vi "Manual.vi"(6 "Cluster":T8={"VISA resource name"="", "baud rate "=9600}, 7 "vi reference":refnum<vi>, 8 "error in (no error)":errorcluster, 9 "IOList_280":T1, 11 "Manual":T4(tab)) -> (0 "error out":errorcluster, 3 "Out reference":refnum<vi>)   [LabVIEW 2015]
uses:
  Control Button/Exit.ctl
  Control Button/Scanner config.ctl
  Galobal variable_TI.vi
  <vilib>/Instr/_visa.llb/VISA Configure Serial Port (Instr).vi
panel:
  out "Z Dir Dn":bool
  out "Z dir Up":bool
  out "Screw SlideFWD":bool
  out "Screw SlideRev":bool
  out "Array":string[](array[string])
  out "Byte Lenth":i32
  out "error out 2":errorcluster
  in  "Stop":T2
  out "NewVal":T3
  in  "Digital Output":T5
  out "LVDT":string
  out "Digital Input":T6
  out "Error Message":string
  out "Dist. data":dbl[](array[numeric]) format="%0.03f"
  out "Error Status":bool
  in  "Scanner config":T7
  out "Read data":string
  out "Boolean":bool
  # "Instruction for Servo motor Operate\n(1)  Switch  ON -OFF  of Fixture Slide servo Brake ON Cmd (P0.19)  \n      from Digital Output tab.\n(2) Switch  ON -OFF  of Fixture Slide Servo Direction Command (P0.20)\n      from Digital Output tab."
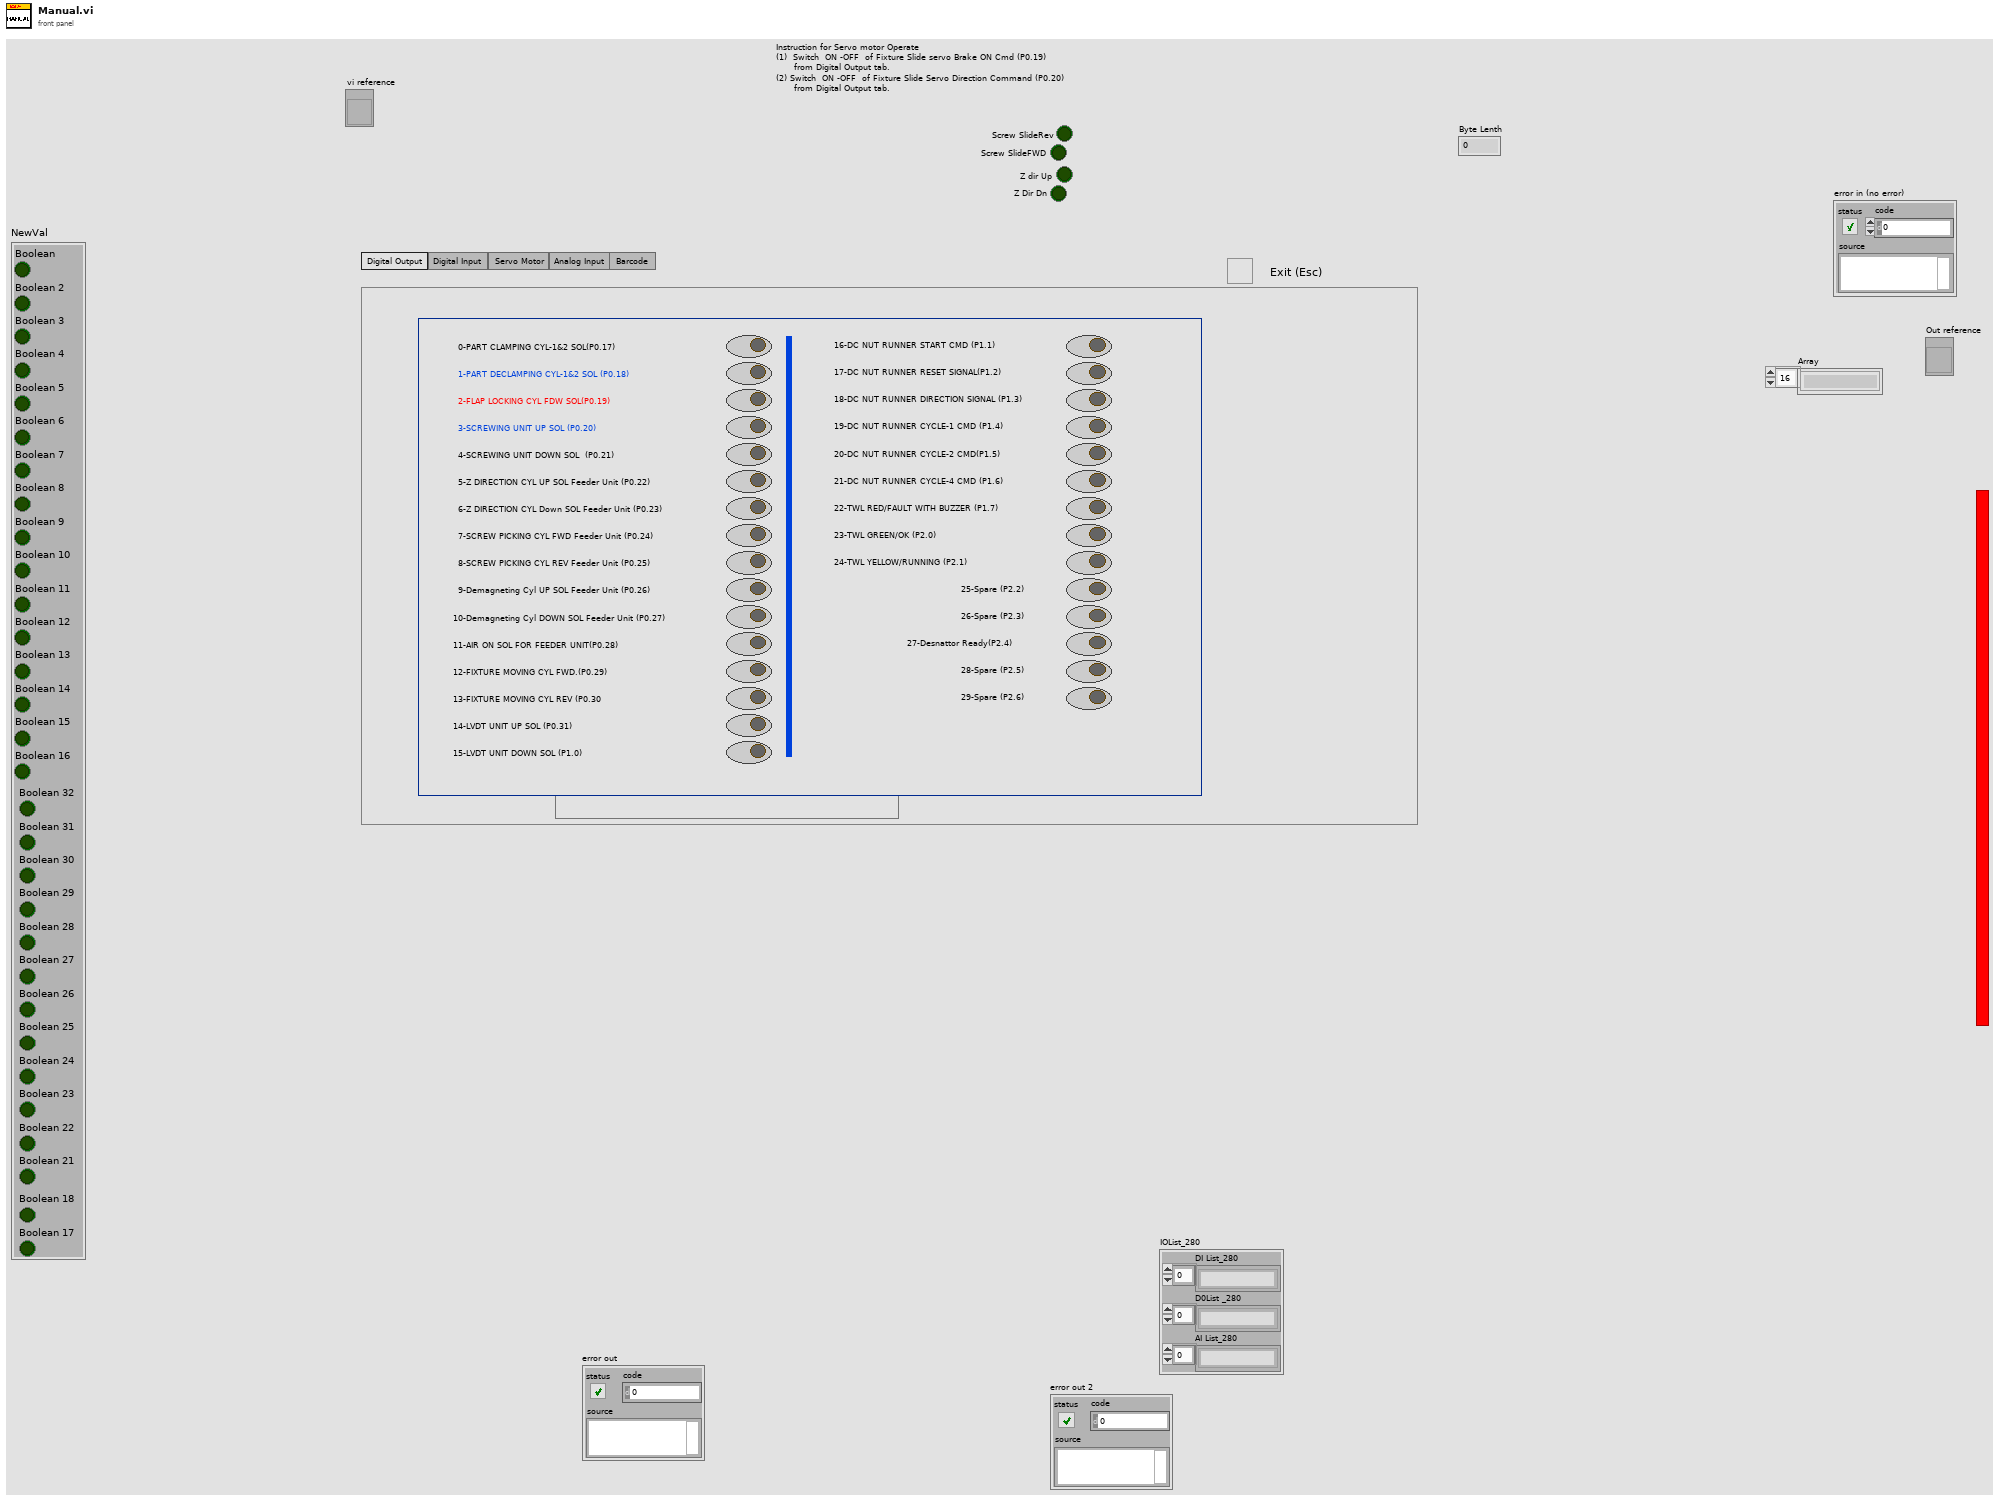
[diagram p1: front panel]
types:
  T1 = cluster{"DI List_280":string[], "D0List _280":string[], "AI List_280":string[]}
  T2 = typedef "Exit.ctl" = bool
  T3 = cluster{"Boolean":bool, "Boolean 2":bool, "Boolean 3":bool, "Boolean 4":bool, "Boolean 5":bool, "Boolean 6":bool, "Boolean 7":bool, "Boolean 8":bool, "Boolean 9":bool, "Boolean 10":bool, "Boolean 11":bool, "Boolean 12":bool, "Boolean 13":bool, "Boolean 14":bool, "Boolean 15":bool, "Boolean 16":bool, "Boolean 17":bool, "Boolean 18":bool, "Boolean 21":bool, "Boolean 22":bool, "Boolean 23":bool, "Boolean 24":bool, "Boolean 25":bool, "Boolean 26":bool, "Boolean 27":bool, "Boolean 28":bool, "Boolean 29":bool, "Boolean 30":bool, "Boolean 31":bool, "Boolean 32":bool}
  T4 = enum32{"Digital Output", "Digital Input", "Servo Motor ", "Analog Input", "Barcode "}
  T5 = cluster{"DO.00":bool, "DO.01":bool, "DO.02":bool, "DO.03":bool, "DO.04":bool, "DO.05":bool, "DO.06":bool, "DO.06":bool, "DO.07":bool, "DO.08":bool, "DO.09":bool, "DO.10":bool, "DO.11":bool, "DO.12":bool, "DO.13":bool, "DO.14":bool, "DO.07 2":bool, "DO.08 2":bool, "DO.09 2":bool, "DO.10 2":bool, "DO.11 2":bool, "DO.12 2":bool, "DO.13 2":bool, "DO.14 2":bool, "DO.00 2":bool, "DO.01 2":bool, "DO.02 2":bool, "DO.03 2":bool, "DO.06 2":bool, "DO.06 3":bool}
  T6 = cluster{"Digital Input":bool, "Digital Input 2":bool, "Digital Input 3":bool, "Digital Input 4":bool, "Digital Input 5":bool, "Digital Input 6":bool, "Digital Input 7":bool, "Digital Input 8":bool, "Digital Input 9":bool, "Digital Input 10":bool, "Digital Input 11":bool, "Digital Input 12":bool, "Digital Input 13":bool, "Digital Input 14":bool, "Digital Input 15":bool, "Digital Input 16":bool, "Digital Input 17":bool, "Digital Input 18":bool, "Digital Input 19":bool, "Digital Input 20":bool, "Digital Input 21":bool, "Digital Input 22":bool, "Digital Input 23":bool, "Digital Input 24":bool, "Digital Input 25":bool, "Digital Input 26":bool, "Digital Input 27":bool, "Digital Input 28":bool, "Digital Input 29":bool, "Digital Input 30":bool, "Digital Input 31":bool, "Digital Input 32":bool, "Digital Input 33":bool, "Digital Input 34":bool, "Digital Input 35":bool, "Digital Input 36":bool, "Digital Input 37":bool, "Digital Input 38":bool, "Digital Input 39":bool, "Digital Input 40":bool, "Digital Input 41":bool, "Digital Input 42":bool, "Digital Input 43":bool, "Digital Input 44":bool}
  T7 = typedef "Scanner config.ctl" = bool
  T8 = cluster{"VISA resource name":refnum<visa-resource-name>, "baud rate ":u32}
  T9 = cluster{"Emergency_1":bool, "Reset_2":bool, "Air Pressure_4":bool, "Safety Sensor_5":bool, "Safety Sensor_6":bool, "Barcode Rev rs_24":bool, "Clamp fwd rs_21":bool, "Servo Fault":bool, "Home _3":bool}
  T10 = cluster{"Digital input[0]":bool, "Digital input[1]":bool, "Digital input[2]":bool, "Digital input[3]":bool, "Digital input[4]":bool, "Digital input[5]":bool, "Digital input[6]":bool, "Digital input[7]":bool, "Digital input[8]":bool, "Digital input[9]":bool, "Digital input[10]":bool, "Digital input[11]":bool, "Digital input[12]":bool, "Digital input[13]":bool, "Digital input[14]":bool, "Digital input[15]":bool, "Digital input[16]":bool, "Digital input[17]":bool, "Digital input[18]":bool, "Digital input[19]":bool, "Digital input[20]":bool, "Digital input[21]":bool, "Digital input[22]":bool, "Digital input[23]":bool, "Digital input[24]":bool, "Digital input[25]":bool, "Digital input[26]":bool, "Digital input[27]":bool, "Digital input[28]":bool, "Digital input[29]":bool, "Digital input[30]":bool, "Digital input[31]":bool, "Digital input[32]":bool, "Digital input[33]":bool, "Digital input[34]":bool, "Digital input[35]":bool, "Digital input[36]":bool, "Digital input[37]":bool, "Digital input[38]":bool, "Digital input[39]":bool, "Digital input[40]":bool, "Digital input[41]":bool, "Digital input[42]":bool, "Digital input[43]":bool}
  T11 = enum16{"Z Dir Up  Screw Slide Rev Cyl_Ddir Dn & Up", "Z Dir Dn Cyl Screw Slide Fwd Cyl"}
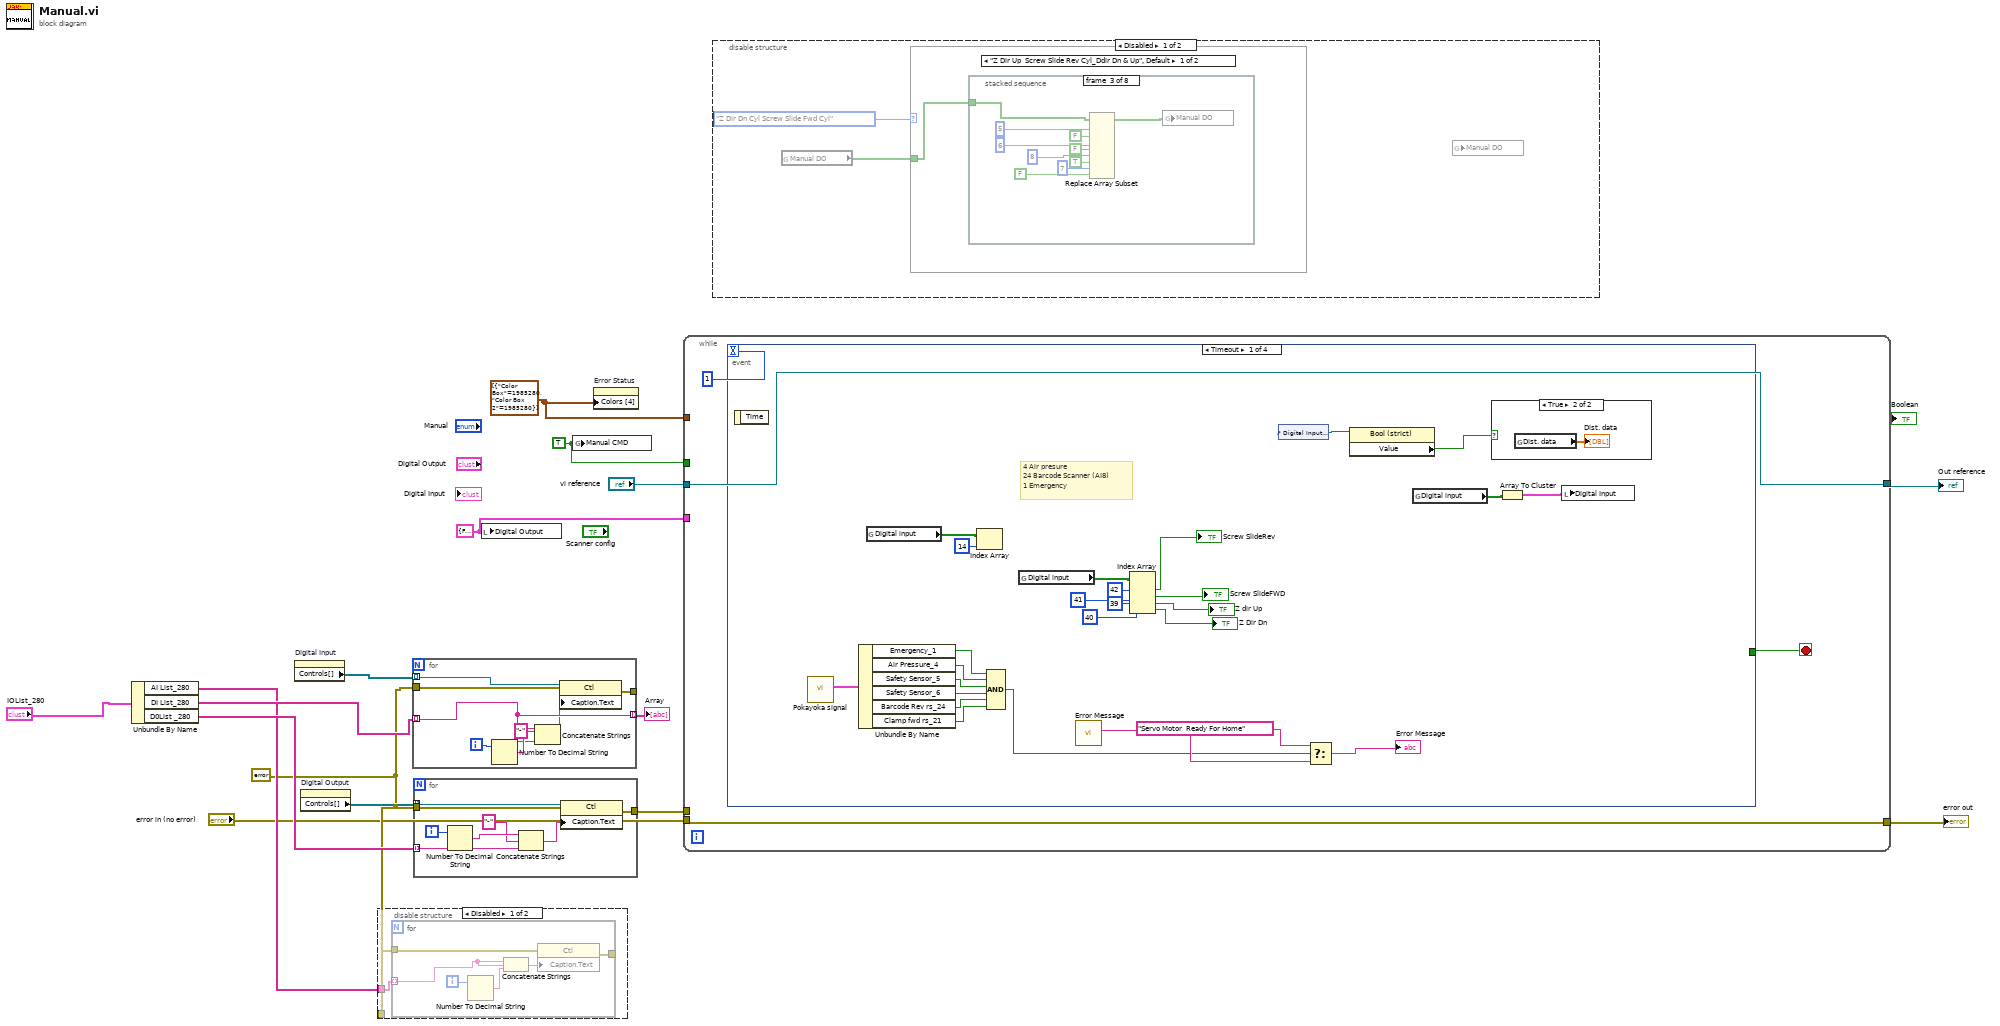
[diagram p0: block diagram]
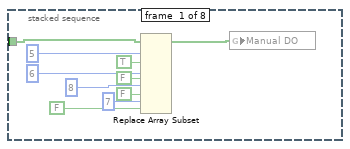
[diagram p2: hidden frame]
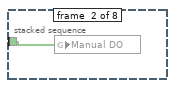
[diagram p3: hidden frame]
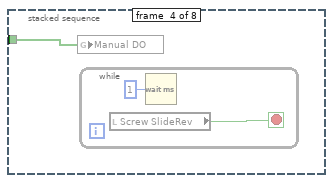
[diagram p4: hidden frame]
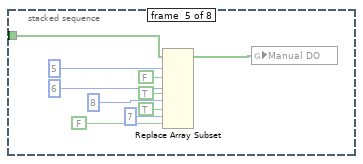
[diagram p5: hidden frame]
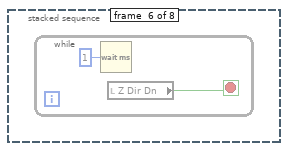
[diagram p6: hidden frame]
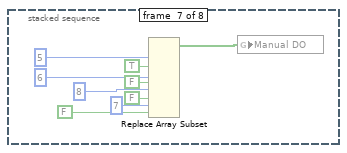
[diagram p7: hidden frame]
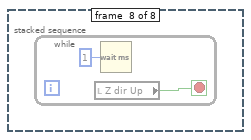
[diagram p8: hidden frame]
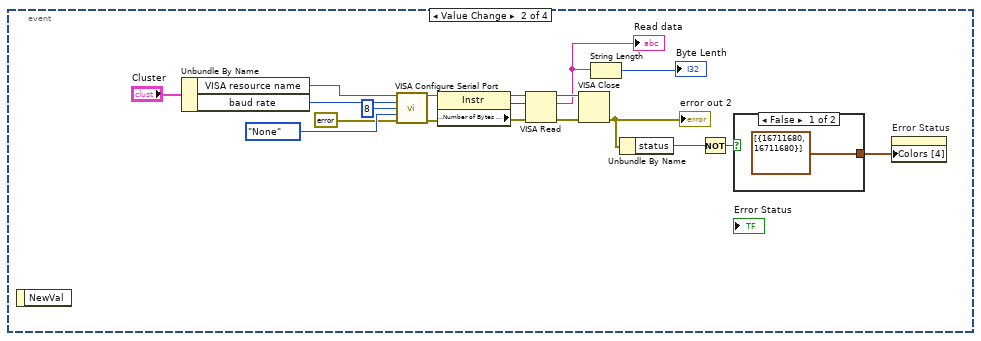
[diagram p13: hidden frame]
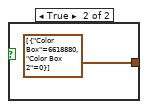
[diagram p14: hidden frame]
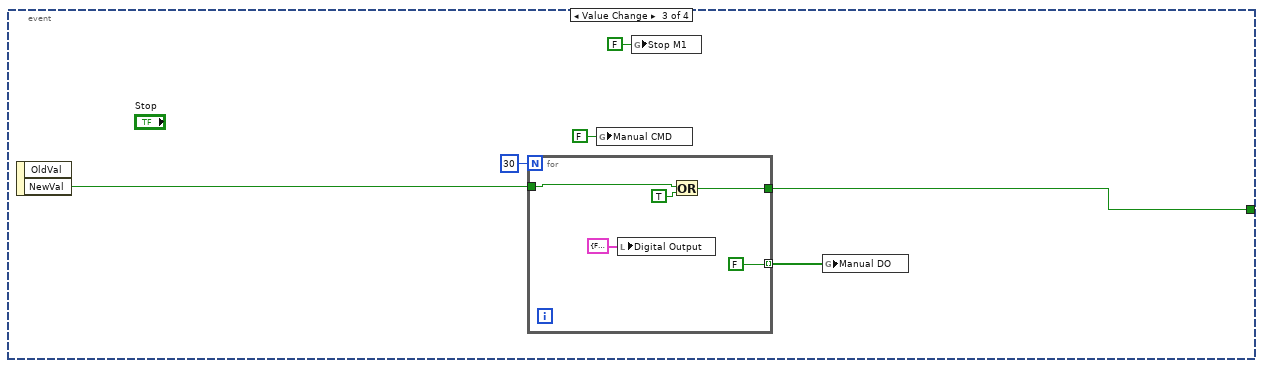
[diagram p15: hidden frame]
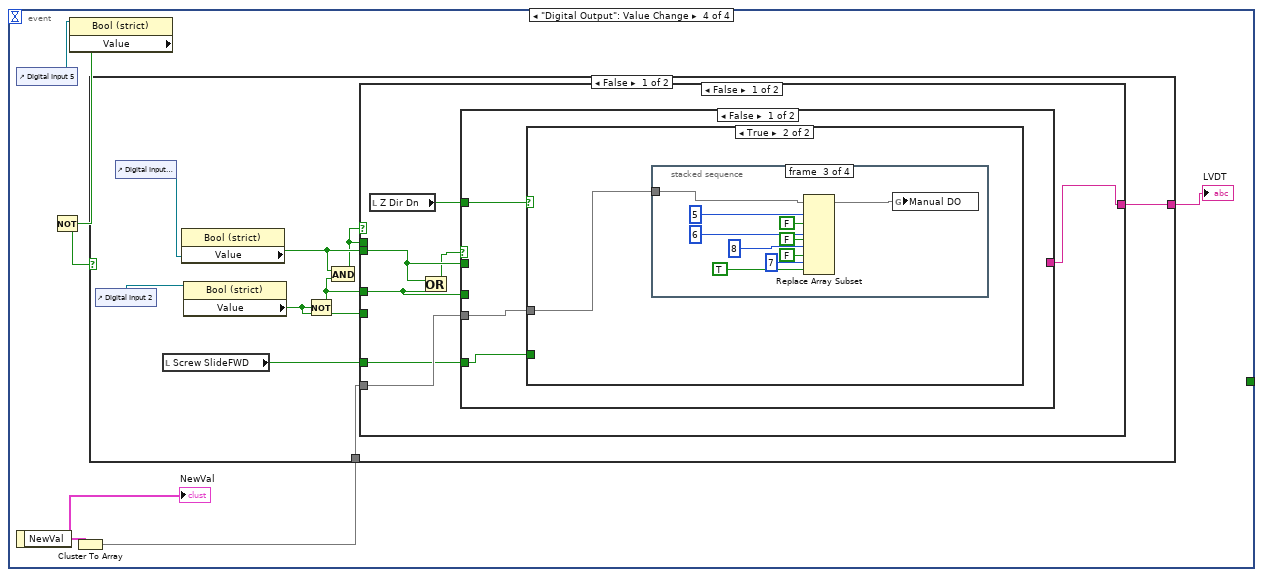
[diagram p16: hidden frame]
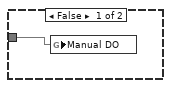
[diagram p17: hidden frame]
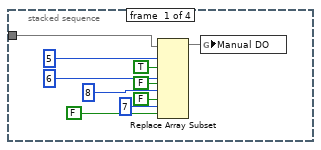
[diagram p18: hidden frame]
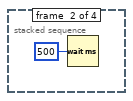
[diagram p19: hidden frame]
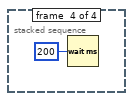
[diagram p20: hidden frame]
diagram:
  w1 = T5 {"DO.00"=FALSE, "DO.01"=FALSE, "DO.02"=FALSE, "DO.03"=FALSE, "DO.04"=FALSE, "DO.05"=FALSE, "DO.06"=FALSE, "DO.06"=FALSE, "DO.07"=FALSE, "DO.08"=FALSE, "DO.09"=FALSE, "DO.10"=FALSE, "DO.11"=FALSE, "DO.12"=FALSE, "DO.13"=FALSE, "DO.14"=FALSE, "DO.07 2"=FALSE, "DO.08 2"=FALSE, "DO.09 2"=FALSE, "DO.10 2"=FALSE, "DO.11 2"=FALSE, "DO.12 2"=FALSE, "DO.13 2"=FALSE, "DO.14 2"=FALSE, "DO.00 2"=FALSE, "DO.01 2"=FALSE, "DO.02 2"=FALSE, "DO.03 2"=FALSE, "DO.06 2"=FALSE, "DO.06 3"=FALSE} ("Digital Output")
  w4 = errorcluster {"status"=FALSE, "code"=0, "source"=""} ("error in (no error)")
  w7 = cluster{"Color Box":u32, "Color Box 2":u32}[] [{"Color Box"=1985280, "Color Box 2"=1985280}] ("Colors [4]")
  w12 = TRUE ("Manual CMD")
  n1 = Unbundle By Name("IOList_280") -> ("AI List_280"=w8:string[], "DI List_280"=w9:string[], "D0List _280"=w11:string[])
  n2 = property on="Digital Input" class="Clust (strict)"() -> ("Controls[]"=w10:refnum<vi>[])  [unwired: 2 in, 2 out]
  n3 = property on="Digital Output" class="Clust (strict)"() -> ("Controls[]"=w15:refnum<vi>[])  [unwired: 2 in, 2 out]
  n4 = disable-structure shown="Disabled" {
    disable-tunnel: w8 -> [w18 _]
    disable-tunnel: w4 -> [w17 _]
    frame Disabled {
      n5 = for {
        tunnel: [w22] -> _
        tunnel: w17 -> [w20]
        tunnel: w18 -> [w19] mode=indexing
        i -> [w23]
        n6 = Number To Decimal String(number=w23) -> (decimal integer string=w21:string)  [unwired: 1 in]
        n7 = Concatenate Strings(w19, w21) -> ()  [unwired: 1 out]
        n8 = property class="Ctl"(error in=w20, "Caption.Text"=w19) -> (error out=w22:errorcluster)  [unwired: 1 in, 1 out]
      }
    }
    frame Enabled {
    }
  }
  n9 = for {
    tunnel: w10 -> [w31] mode=indexing
    tunnel: [w29] -> _
    tunnel: w4 -> [w28]
    tunnel: w9 -> [w25] mode=indexing
    tunnel: [w25] -> w5 mode=indexing
    i -> [w30]
    n10 = Number To Decimal String(number=w30) -> (decimal integer string=w27:string)  [unwired: 1 in]
    n11 = Concatenate Strings(w27, "-" ("string"), w25) -> (w24:string)
    n12 = property class="Ctl"(reference=w31, error in=w28, "Caption.Text"=w24) -> (error out=w29:errorcluster)  [unwired: 1 out]
  }
  "Array" <- w5
  n13 = for {
    tunnel: w15 -> [w39] mode=indexing
    tunnel: [w37] -> w16
    tunnel: w4 -> [w36]
    tunnel: w11 -> [w33] mode=indexing
    i -> [w38]
    n14 = Number To Decimal String(number=w38) -> (decimal integer string=w35:string)  [unwired: 1 in]
    n15 = Concatenate Strings(w35, "-" ("string"), w33) -> (w32:string)
    n16 = property class="Ctl"(reference=w39, error in=w36, "Caption.Text"=w32) -> (error out=w37:errorcluster)  [unwired: 1 out]
  }
  n17 = local write "Digital Output"(w1) -> ()
  n18 = global write "Galobal variable_TI.vi" "Manual CMD"(w12) -> ()
  n19 = property on="Error Status" class="Bool (strict)"("Colors [4]"=w7) -> ()  [unwired: 2 in, 2 out]
  n20 = while {
    tunnel: w16 -> [_]
    tunnel: [w41] -> w14
    tunnel: "vi reference" -> [w42]
    tunnel: [w42] -> w13
    tunnel: w12 -> [_]
    tunnel: w7 -> [_]
    tunnel: "error in (no error)" -> [w41]
    tunnel: w1 -> [_]
    stop <- w40 stop-if-true
    n21 = event shown="[0] Timeout" {
      selector: _ -> [_ _ _ _]
      dyn-events: _ -> [_ _ _ _]
      timeout: 1 -> [_ _ _ _]
      tunnel: [_ _ w92 _] -> w40
      event Timeout {
        # "4 Air presure\n24 Barcode Scanner (AI8)\n1 Emergency"
        n22 = event-data() -> ()  [unwired: 1 in, 1 out]
        n23 = call "Pokayoka signal.vi"() -> ("output cluster"=w64:T9)  [unwired: 10 in, 1 out]
        n24 = Unbundle By Name(w64) -> ("Emergency_1"=w57:bool, "Air Pressure_4"=w63:bool, "Safety Sensor_5"=w62:bool, "Safety Sensor_6"=w61:bool, "Barcode Rev rs_24"=w60:bool, "Clamp fwd rs_21"=w59:bool)
        n25 = global read "Galobal variable_TI.vi" "Digital input"() -> (w56:bool[])
        n26 = Index Array(array=w56, index=14) -> ()  [unwired: 1 out]
        n27 = Compound Arithmetic op=AND(w57, w63, w62, w61, w60, w59) -> (w58:bool)
        n28 = global read "Galobal variable_TI.vi" "Digital input"() -> (w53:bool[])
        n29 = call "Error Message.vi"() -> ("Error"=w66:string)  [unwired: 11 in]
        n30 = Index Array(array=w53, index #1=42 ("index"), index #2=41 ("index"), index #3=39 ("index"), index #4=40 ("index")) -> (element #1=→"Screw SlideRev":bool, element #2=→"Screw SlideFWD":bool, element #3=→"Z dir Up":bool, element #4=→"Z Dir Dn":bool)
        n31 = control-ref of="Digital Input 16"() -> (w45:refnum<vi>)
        n32 = Select(t="Servo Motor  Ready For Home", s=w58, f=w66) -> (s? t:f=→"Error Message":string)
        n33 = property class="Bool (strict)"(reference=w45) -> ("Value"=w44:bool)  [unwired: 1 in, 2 out]
        n34 = global read "Galobal variable_TI.vi" "Digital input"() -> (w68:bool[])
        n35 = case shown="True" w44 {
          frame False {
          }
          frame True {
            n36 = global read "Galobal variable_TI.vi" "Dist. data"() -> (→"Dist. data":dbl[])
          }
        }
        n37 = Array To Cluster(array=w68) -> (cluster=w69:T10)
        n38 = local write "Digital Input"(w69) -> ()
      }
      event Value Change {
        n39 = event-data() -> ()  [unwired: 1 in, 1 out]
        n40 = Unbundle By Name("Cluster") -> ("VISA resource name"=w89:refnum<visa-resource-name>, "baud rate"=w88:u32)
        n41 = call-poly "VISA Configure Serial Port"("VISA resource name"=w89, "baud rate (9600)"=w88, "data bits (8)"=u16 8, "parity (0:none)"=enum16{"None", "Odd", "Even", "Mark", "Space"}."None", "error in (no error)"=errorcluster {"status"=FALSE, "code"=0, "source"=""} ("error in (no error) 2")) -> ("VISA resource name out"=w87:refnum<visa-resource-name>, "error out"=w85:errorcluster)  [unwired: 9 in]
        n42 = property class="Instr"(reference=w87, error in=w85) -> (reference out=w86:refnum<visa-resource-name>, error out=w84:errorcluster, "Serial Settings:Number of Bytes at Serial Port"=w83:u32)
        n43 = VISA Read(VISA resource name=w86, byte count=w83, error in (no error)=w84) -> (VISA resource name out=w81:refnum<visa-resource-name>, read buffer=w79:string, error out=w80:errorcluster)  [unwired: 1 out]
        "Read data" <- w79
        n44 = VISA Close(VISA resource name=w81, error in (no error)=w80) -> (error out=w77:errorcluster)
        "error out 2" <- w77
        n45 = String Length(string=w79) -> (length=→"Byte Lenth":i32)
        n46 = Unbundle By Name(w77) -> ("status"=w76:bool)
        n47 = Not(x=w76) -> (.not. x?=w74:bool)
        n48 = case shown="False" w74 {
          tunnel: [cluster{"Color Box":u32, "Color Box 2":u32}[] [{"Color Box"=16711680, "Color Box 2"=16711680}] ("Colors [4]") cluster{"Color Box":u32, "Color Box 2":u32}[] [{"Color Box"=6618880, "Color Box 2"=0}] ("Colors [4]")] -> w75
          frame False {
          }
          frame True {
          }
        }
        n49 = property on="Error Status" class="Bool (strict)"("Colors [4]"=w75) -> ()  [unwired: 2 in, 2 out]
      }
      event Value Change {
        n50 = event-data() -> ("NewVal"=w93:T2)  [unwired: 1 in, 1 out]
        n51 = for {
          N: 30 -> [_]
          tunnel: [FALSE] -> w95 mode=indexing
          tunnel: w93 -> [w100]
          tunnel: [w99] -> w92
          n52 = local write "Digital Output"(T5 {"DO.00"=FALSE, "DO.01"=FALSE, "DO.02"=FALSE, "DO.03"=FALSE, "DO.04"=FALSE, "DO.05"=FALSE, "DO.06"=FALSE, "DO.06"=FALSE, "DO.07"=FALSE, "DO.08"=FALSE, "DO.09"=FALSE, "DO.10"=FALSE, "DO.11"=FALSE, "DO.12"=FALSE, "DO.13"=FALSE, "DO.14"=FALSE, "DO.07 2"=FALSE, "DO.08 2"=FALSE, "DO.09 2"=FALSE, "DO.10 2"=FALSE, "DO.11 2"=FALSE, "DO.12 2"=FALSE, "DO.13 2"=FALSE, "DO.14 2"=FALSE, "DO.00 2"=FALSE, "DO.01 2"=FALSE, "DO.02 2"=FALSE, "DO.03 2"=FALSE, "DO.06 2"=FALSE, "DO.06 3"=FALSE} ("Digital Output")) -> ()
          n53 = Or(x=w100, y=TRUE) -> (x .or. y?=w99:T2)
        }
        n54 = global write "Galobal variable_TI.vi" "Manual CMD"(FALSE ("Manual CMD")) -> ()
        n55 = global write "Galobal variable_TI.vi" "Stop M1"(FALSE ("Stop M1")) -> ()
        n56 = global write "Galobal variable_TI.vi" "Manual DO"(w95) -> ()
      }
      event "Digital Output": Value Change {
        n57 = control-ref of="Digital Input 5"() -> (w105:refnum<vi>)
        n58 = event-data() -> ("NewVal"=w107:T5)  [unwired: 1 in]
        "NewVal" <- w107
        n59 = property class="Bool (strict)"(reference=w105) -> ("Value"=w104:bool)  [unwired: 1 in, 2 out]
        n60 = Not(x=w104) -> (.not. x?=w103:bool)
        n61 = Cluster To Array(cluster=w107) -> (array=w108:bool[])
        n62 = case shown="False" w103 {
          tunnel: w108 -> [w117 _]
          tunnel: [w109 _] -> w106
          frame False {
            n63 = control-ref of="Digital Input 2"() -> (w115:refnum<vi>)
            n64 = control-ref of="Digital Input 16"() -> (w116:refnum<vi>)
            n65 = local read "Screw SlideFWD"() -> (w110:bool)
            n66 = property class="Bool (strict)"(reference=w116) -> ("Value"=w114:bool)  [unwired: 1 in, 2 out]
            n67 = property class="Bool (strict)"(reference=w115) -> ("Value"=w112:bool)  [unwired: 1 in, 2 out]
            n68 = Not(x=w112) -> (.not. x?=w113:bool)
            n69 = And(x=w114, y=w113) -> (x .and. y?=w111:bool)
            n70 = case shown="False" w111 {
              tunnel: [w124 _] -> w109
              tunnel: w117 -> [w121 w196]
              tunnel: w114 -> [w123 w197]
              tunnel: w113 -> [w120 _]
              tunnel: w112 -> [_ _]
              tunnel: w111 -> [_ _]
              tunnel: w110 -> [w119 _]
              frame False {
                n71 = local read "Z Dir Dn"() -> (w118:bool)
                n72 = Or(x=w123, y=w120) -> (x .or. y?=w122:bool)
                n73 = case shown="False" w122 {
                  tunnel: w123 -> [_ w153]
                  tunnel: [_ w155] -> w124
                  tunnel: w121 -> [w127 w154]
                  tunnel: w120 -> [_ w152]
                  tunnel: w119 -> [w126 _]
                  tunnel: w118 -> [w125 _]
                  frame False {
                    n74 = case shown="True" w125 {
                      tunnel: w127 -> [w128 w129]
                      tunnel: w126 -> [_ _]
                      frame False {
                        n75 = global write "Galobal variable_TI.vi" "Manual DO"(w128) -> ()
                      }
                      frame True {
                        n76 = stacked-sequence {
                          tunnel: w129 -> [w131 _ w141 _]
                          frame #0 {
                            n77 = Replace Array Subset(array=w131, new element #1=TRUE ("new element/subarray"), index #1=5 ("index"), new element #2=FALSE ("new element/subarray"), index #2=6 ("index"), new element #3=FALSE ("new element/subarray"), index #3=8 ("index"), new element #4=FALSE ("new element/subarray"), index #4=7 ("index")) -> (w130:bool[])
                            n78 = global write "Galobal variable_TI.vi" "Manual DO"(w130) -> ()
                          }
                          frame #1 {
                            n79 = Wait (ms)(milliseconds to wait=u32 500) -> ()  [unwired: 1 out]
                          }
                          frame #2 {
                            n80 = Replace Array Subset(array=w141, new element #1=FALSE ("new element/subarray"), index #1=5 ("index"), new element #2=FALSE ("new element/subarray"), index #2=6 ("index"), new element #3=FALSE ("new element/subarray"), index #3=8 ("index"), new element #4=TRUE ("new element/subarray"), index #4=7 ("index")) -> (w146:bool[])
                            n81 = global write "Galobal variable_TI.vi" "Manual DO"(w146) -> ()
                          }
                          frame #3 {
                            n82 = Wait (ms)(milliseconds to wait=u32 200) -> ()  [unwired: 1 out]
                          }
                        }
                      }
                    }
                  }
                  frame True {
                    n83 = case shown="False" w153 {
                      tunnel: w153 -> [_ _]
                      tunnel: [w159 _] -> w155
                      tunnel: w154 -> [w156 w190]
                      tunnel: w152 -> [w158 _]
                      frame False {
                        n84 = local read "Z Dir Dn"() -> (w157:bool)
                        n85 = case shown="True" w157 {
                          tunnel: [w161 _] -> w159
                          tunnel: w158 -> [w160 _]
                          tunnel: w156 -> [_ w164]
                          frame False {
                            n86 = Select(t="LVDT  DN RS _P0.14", s=w160, f="Emergency") -> (s? t:f=w161:string)
                          }
                          frame True {
                            n87 = stacked-sequence {
                              tunnel: w164 -> [w166 _ w176]
                              frame #0 {
                                n88 = Replace Array Subset(array=w166, new element #1=TRUE ("new element/subarray"), index #1=5 ("index"), new element #2=FALSE ("new element/subarray"), index #2=6 ("index"), new element #3=FALSE ("new element/subarray"), index #3=8 ("index"), new element #4=FALSE ("new element/subarray"), index #4=7 ("index")) -> (w165:bool[])
                                n89 = global write "Galobal variable_TI.vi" "Manual DO"(w165) -> ()
                              }
                              frame #1 {
                                n90 = Wait (ms)(milliseconds to wait=u32 100) -> ()  [unwired: 1 out]
                              }
                              frame #2 {
                                n91 = Replace Array Subset(array=w176, new element #1=FALSE ("new element/subarray"), index #1=5 ("index"), new element #2=FALSE ("new element/subarray"), index #2=6 ("index"), new element #3=FALSE ("new element/subarray"), index #3=8 ("index"), new element #4=TRUE ("new element/subarray"), index #4=7 ("index")) -> (w181:bool[])
                                n92 = global write "Galobal variable_TI.vi" "Manual DO"(w181) -> ()
                              }
                            }
                          }
                        }
                      }
                      frame True {
                        n93 = Replace Array Subset(array=w190, new element #1=FALSE ("new element/subarray"), index #1=12 ("index"), new element #2=FALSE ("new element/subarray"), index #2=13 ("index"), new element #3=TRUE ("new element/subarray"), index #3=14 ("index"), new element #4=FALSE ("new element/subarray"), index #4=15 ("index")) -> (w191:bool[])
                        n94 = global write "Galobal variable_TI.vi" "Manual DO"(w191) -> ()
                      }
                    }
                  }
                }
              }
              frame True {
                n95 = case shown="True" w197 {
                  tunnel: w197 -> [_ _]
                  tunnel: w196 -> [_ w207]
                  frame False {
                  }
                  frame True {
                    n96 = Replace Array Subset(array=w207, new element #1=FALSE ("new element/subarray"), index #1=15 ("index"), new element #2=TRUE ("new element/subarray"), index #2=14 ("index"), new element #3=FALSE ("new element/subarray"), index #3=12 ("index"), new element #4=FALSE ("new element/subarray"), index #4=13 ("index")) -> (w206:bool[])
                    n97 = global write "Galobal variable_TI.vi" "Manual DO"(w206) -> ()
                  }
                }
              }
            }
          }
          frame True {
          }
        }
        "LVDT" <- w106
      }
    }
  }
  "error out" <- w14
  "Out reference" <- w13
  n98 = disable-structure shown="Disabled" {
    frame Disabled {
      n99 = global read "Galobal variable_TI.vi" "Manual DO"() -> (w208:bool[])
      n100 = case shown="\"Z Dir Up  Screw Slide Rev Cyl_Ddir Dn & Up\", Default" T11."Z Dir Dn Cyl Screw Slide Fwd Cyl" {
        tunnel: w208 -> [w210 _]
        frame "Z Dir Up  Screw Slide Rev Cyl_Ddir Dn & Up", Default {
          n101 = stacked-sequence {
            tunnel: w210 -> [w211 w221 w222 w232 w235 _ _ _]
            frame #0 {
              n102 = Replace Array Subset(array=w211, new element #1=TRUE ("new element/subarray"), index #1=5 ("index"), new element #2=FALSE ("new element/subarray"), index #2=6 ("index"), new element #3=FALSE ("new element/subarray"), index #3=8 ("index"), new element #4=FALSE ("new element/subarray"), index #4=7 ("index")) -> (w216:bool[])
              n103 = global write "Galobal variable_TI.vi" "Manual DO"(w216) -> ()
            }
            frame #1 {
              n104 = global write "Galobal variable_TI.vi" "Manual DO"(w221) -> ()
            }
            frame #2 {
              n105 = Replace Array Subset(array=w222, new element #1=FALSE ("new element/subarray"), index #1=5 ("index"), new element #2=FALSE ("new element/subarray"), index #2=6 ("index"), new element #3=TRUE ("new element/subarray"), index #3=8 ("index"), new element #4=FALSE ("new element/subarray"), index #4=7 ("index")) -> (w227:bool[])
              n106 = global write "Galobal variable_TI.vi" "Manual DO"(w227) -> ()
            }
            frame #3 {
              n107 = global write "Galobal variable_TI.vi" "Manual DO"(w232) -> ()
              n108 = while {
                stop <- w233 stop-if-true
                n109 = local read "Screw SlideRev"() -> (w233:bool)
                n110 = Wait (ms)(milliseconds to wait=u32 1) -> ()  [unwired: 1 out]
              }
            }
            frame #4 {
              n111 = Replace Array Subset(array=w235, new element #1=FALSE ("new element/subarray"), index #1=5 ("index"), new element #2=TRUE ("new element/subarray"), index #2=6 ("index"), new element #3=TRUE ("new element/subarray"), index #3=8 ("index"), new element #4=FALSE ("new element/subarray"), index #4=7 ("index")) -> (w240:bool[])
              n112 = global write "Galobal variable_TI.vi" "Manual DO"(w240) -> ()
            }
            frame #5 {
              n113 = while {
                stop <- w245 stop-if-true
                n114 = Wait (ms)(milliseconds to wait=u32 1) -> ()  [unwired: 1 out]
                n115 = local read "Z Dir Dn"() -> (w245:bool)
              }
            }
            frame #6 {
              n116 = Replace Array Subset(new element #1=TRUE ("new element/subarray"), index #1=5 ("index"), new element #2=FALSE ("new element/subarray"), index #2=6 ("index"), new element #3=FALSE ("new element/subarray"), index #3=8 ("index"), new element #4=FALSE ("new element/subarray"), index #4=7 ("index")) -> (w251:bool[])  [unwired: 1 in]
              n117 = global write "Galobal variable_TI.vi" "Manual DO"(w251) -> ()
            }
            frame #7 {
              n118 = while {
                stop <- w257 stop-if-true
                n119 = local read "Z dir Up"() -> (w257:bool)
                n120 = Wait (ms)(milliseconds to wait=u32 1) -> ()  [unwired: 1 out]
              }
            }
          }
        }
        frame "Z Dir Dn Cyl Screw Slide Fwd Cyl" {
        }
      }
      n121 = global read "Galobal variable_TI.vi" "Manual DO"() -> ()  [unwired: 1 in]
    }
    frame Enabled {
    }
  }
